vi "SLSC Create VS Channels for subVI.vi"() -> (3 "Outgoing configuration":T3(array[cluster]))   [LabVIEW 2015, in "SLSC-12201 DIO System Explorer.lvlib"]
uses:
  SLSC-12201 DIO System Explorer.lvlib
  <vilib>/NI Veristand/Custom Device API/Custom Device Channel.ctl
  <vilib>/NI Veristand/Custom Device API/Custom Device Channel Type.ctl
  <vilib>/NI Veristand/Custom Device API/Custom Device API.lvlib
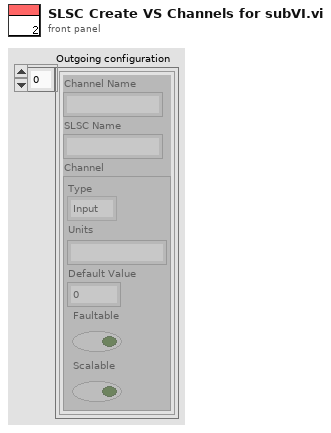
[diagram p1: front panel]
types:
  T1 = typedef "Custom Device API.lvlib/Custom Device Channel.ctl" = cluster{"Type":T2, "Units":string, "Default Value":dbl, "Faultable":bool, "Scalable":bool}
  T2 = typedef "Custom Device API.lvlib/Custom Device Channel Type.ctl" = enum16{"Input", "Output"}
  T3 = cluster{"Channel Name":string, "SLSC Name":string, "Channel":T1}[]
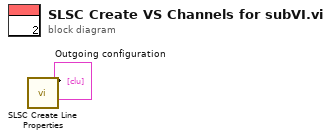
[diagram p0: block diagram]
diagram:
  n1 = call "SLSC Create Line Properties.vi"() -> ("Outgoing configuration"=→"Outgoing configuration":T3)  [unwired: 11 in]
